vi "video.create_commit.vi"(8 "error in":errorcluster, 11 "VideoCreateStaging in":refnum<class "VideoCreateStaging.lvclass">) -> (0 "error out":errorcluster, 2 "Video":refnum<class "Video.lvclass">, 3 "VideoCreateStaging out":refnum<class "VideoCreateStaging.lvclass">)   [LabVIEW 2020, in "VideoCreateStaging.lvclass"]
doc: "Creates the staged video in Nominal and returns a handle to it."
uses:
  VideoCreateStaging.lvclass
  VideoCreateStaging.lvclass/VideoCreateStaging.ctl
  client.lvlib
  Video/Video.lvclass
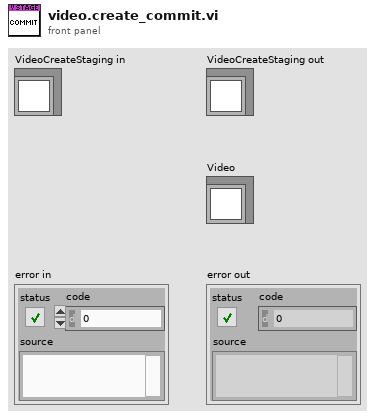
[diagram p1: front panel]
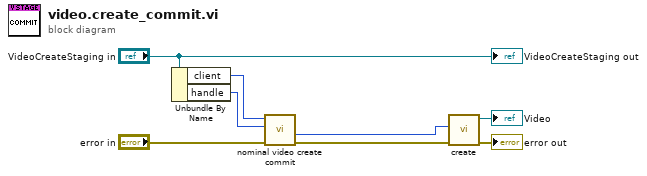
[diagram p0: block diagram]
diagram:
  n1 = Unbundle By Name("VideoCreateStaging in") -> ("client"=w7:i32, "handle"=w5:i32)
  n2 = call "nominal video create commit.vi"("error in (no error)"="error in", "staging"=w5, "client"=w7) -> ("error out"=w2:errorcluster, "out_video out"=w3:i32)  [unwired: 6 in, 1 out]
  n3 = call "create.vi"("error in (no error)"=w2, "handle"=w3) -> ("error out"=→"error out":errorcluster, "Video"=→"Video":refnum<class "Video.lvclass">)  [unwired: 8 in]
  "VideoCreateStaging out" <- "VideoCreateStaging in"
